vi "Get ControlMode.vi"(8 "error in":errorcluster, 11 "VISA resource name in":refnum<visa-resource-name>) -> (0 "error out":errorcluster, 1 "Control (out)":enum16{"Internal", "External"}(ring), 3 "VISA resource name out":refnum<visa-resource-name>)   [LabVIEW 2018, in "JULABO DeviceDriver.lvlib"]
doc: "This VI returns the status (internal, 0 or external, 1) to indicate the type of control, that is actually used. \n\nNote:\nThis function is not available for devices which do not have an external sensor plug."
uses:
  JULABO DeviceDriver.lvlib
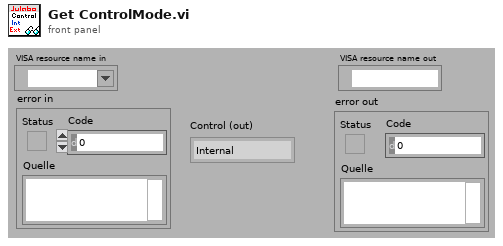
[diagram p1: front panel]
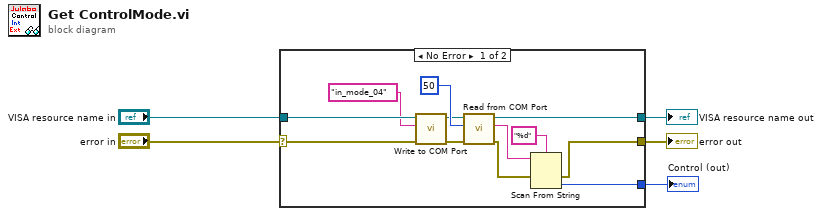
[diagram p0: block diagram]
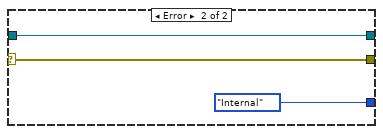
[diagram p2: hidden frame]
diagram:
  n1 = case shown="No Error" "error in" {
    selector: "error in" -> [w14 w19]
    tunnel: [w17 w20] -> w5
    tunnel: "VISA resource name in" -> [w16 w20]
    tunnel: [w15 w19] -> w3
    tunnel: [w6 enum16{"Internal", "External"}."Internal" ("Control (out)")] -> w1
    frame No Error {
      n2 = call "Write to COM Port.vi"("error in"=w14, "Command (input)"="in_mode_04", "VISA resource name in"=w16) -> ("error out"=w8:errorcluster, "VISA resource name out"=w9:refnum<visa-resource-name>)  [unwired: 7 in]
      n3 = call "Read from COM Port.vi"("error in"=w8, "Byte to Read (-1:All)"=u32 50 ("Anzahl der Byte"), "VISA resource name in"=w9) -> ("error out"=w7:errorcluster, "String (output)"=w11:string, "VISA resource name out"=w17:refnum<visa-resource-name>)  [unwired: 5 in, 1 out]
      n4 = Scan From String(format string="%d" ("Format-String"), input string=w11, error in=w7) -> (error out=w15:errorcluster, output 1=w6:i32)  [unwired: 2 in, 2 out]
    }
    frame Error {
    }
  }
  "error out" <- w3
  "VISA resource name out" <- w5
  "Control (out)" <- w1
